vi "Parsing_TheGoodOne.vi"(7 "Search_Params":string[](array[string])=["x1", "y1", "z1", "x2", "y2", "z2"], 11 "Input":string) -> (3 "Positions":i32[](array[numeric]))   [LabVIEW 2016]
panel:
  out "Distance2":dbl
  out "Distance1":dbl
  out "Area2":dbl
  out "Area1":dbl
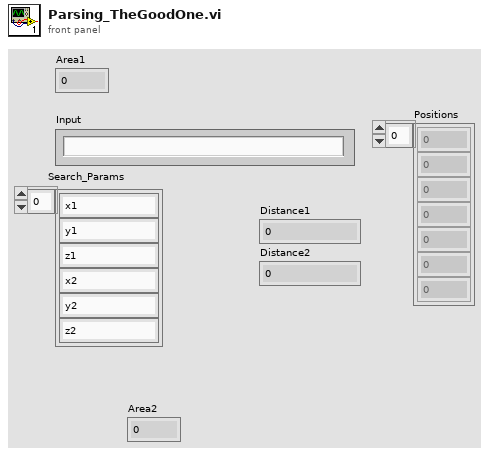
[diagram p1: front panel]
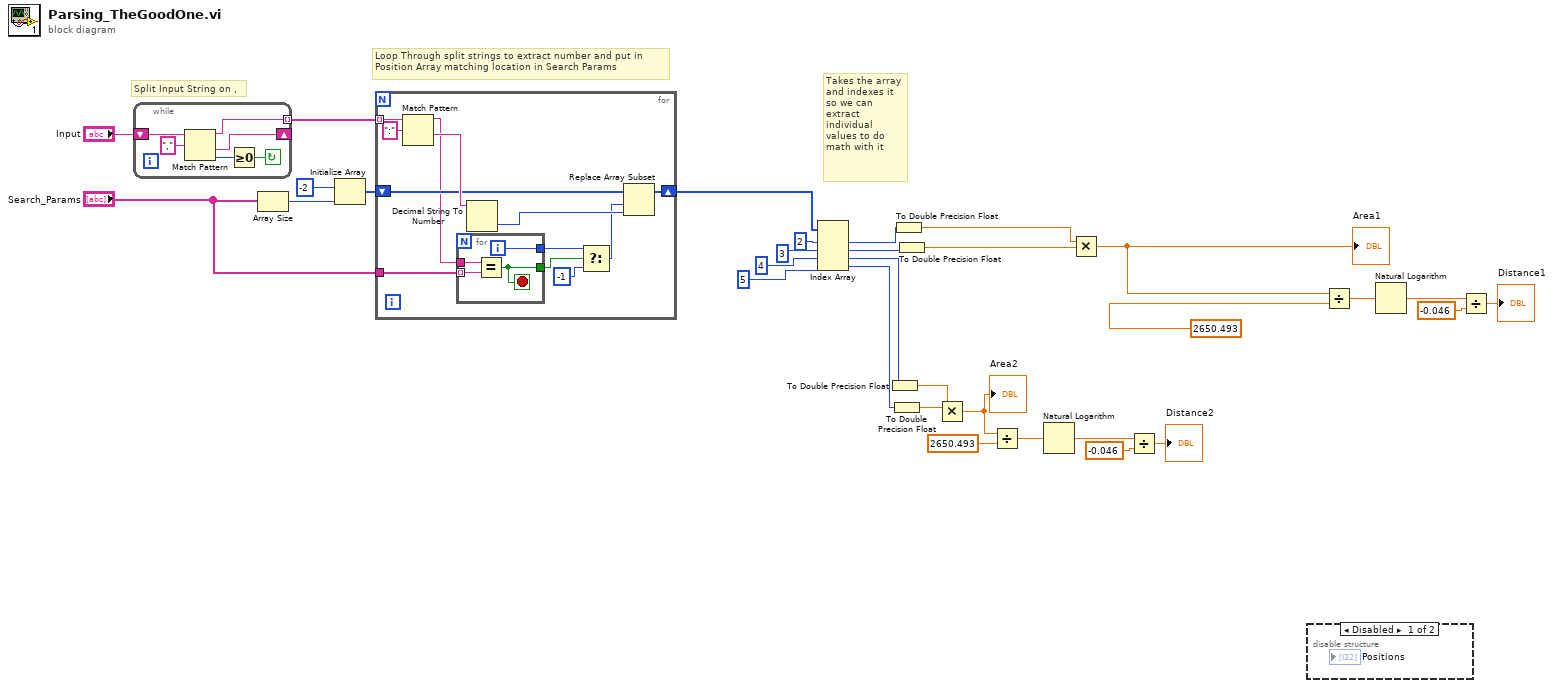
[diagram p0: block diagram]
diagram:
  # "Takes the array and indexes it so we can extract individual values to do math with it"
  # "Loop Through split strings to extract number and put in\nPosition Array matching location in Search Params"
  # "Split Input String on ,"
  n1 = while {
    shift-right: [w34] -> _
    shift-left: "Input" -> [w37]
    tunnel: [w35] -> w30 mode=indexing
    stop <- w32 continue-if-true
    n2 = Match Pattern(string=w37, regular expression=",") -> (before substring=w35:string, after substring=w34:string, offset past match=w33:i32)  [unwired: 1 in, 1 out]
    n3 = Greater Or Equal To 0?(x=w33) -> (x >= 0?=w32:bool)
  }
  n4 = Array Size(array="Search_Params") -> (size(s)=w26:i32)
  n5 = Initialize Array(-2 ("element"), w26) -> (w28:i32[])
  n6 = for {
    tunnel: w30 -> [w49] mode=indexing
    shift-right: [w45] -> w13
    shift-left: w28 -> [w46]
    tunnel: "Search_Params" -> [w42]
    n7 = Match Pattern(string=w49, regular expression=":") -> (before substring=w43:string, after substring=w47:string)  [unwired: 1 in, 2 out]
    n8 = for {
      tunnel: w43 -> [w53]
      tunnel: w42 -> [w52] mode=indexing
      tunnel: [w50] -> w41
      tunnel: [w51] -> w40
      i -> [w51]
      stop <- w50 stop-if-true
      n9 = Equal?(x=w53, y=w52) -> (x = y?=w50:bool)
    }
    n10 = Decimal String To Number(string=w47) -> (number=w44:i32)  [unwired: 2 in, 1 out]
    n11 = Select(t=w40, s=w41, f=-1) -> (s? t:f=w38:i32)
    n12 = Replace Array Subset(array=w46, new element=w44, index=w38) -> (w45:i32[])
  }
  n13 = Index Array(array=w13, index #1=2 ("index"), index #2=3 ("index"), index #3=4 ("index"), index #4=5 ("index")) -> (element #1=w10:i32, element #2=w8:i32, element #3=w5:i32, element #4=w2:i32)
  n14 = To Double Precision Float(number=w5) -> (double precision float=w4:dbl)
  n15 = To Double Precision Float(number=w2) -> (double precision float=w1:dbl)
  n16 = To Double Precision Float(number=w10) -> (double precision float=w9:dbl)
  n17 = To Double Precision Float(number=w8) -> (double precision float=w7:dbl)
  n18 = Multiply(x=w4, y=w1) -> (x*y=w16:dbl)
  "Area2" <- w16
  n19 = Divide(x=w16, y=2650.493) -> (x/y=w18:dbl)
  n20 = Natural Logarithm(1:w18) -> (0:w19:dbl)
  n21 = Multiply(x=w9, y=w7) -> (x*y=w25:dbl)
  "Area1" <- w25
  n22 = Divide(x=w19, y=-0.046) -> (x/y=→"Distance2":dbl)
  n23 = disable-structure shown="Disabled" {
    frame Disabled {
    }
    frame Enabled {
    }
  }
  n24 = Divide(x=w25, y=2650.493) -> (x/y=w23:dbl)
  n25 = Natural Logarithm(1:w23) -> (0:w22:dbl)
  n26 = Divide(x=w22, y=-0.046) -> (x/y=→"Distance1":dbl)
